vi "Moving Average.vi"(10 "Value":bool, 11 "Time Target (s)":dbl=0.25) -> (3 "Moving Boolean Average":bool)   [LabVIEW 2014]
uses:
  <vilib>/Analysis/baseanly.llb/Mean (DBL).vi
  <vilib>/Analysis/NI_AALBase.lvlib
panel:
  out "Elapsed Time (s)":dbl=0.3622617721557617
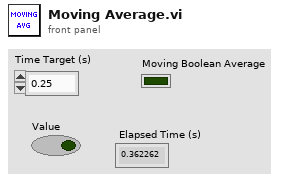
[diagram p1: front panel]
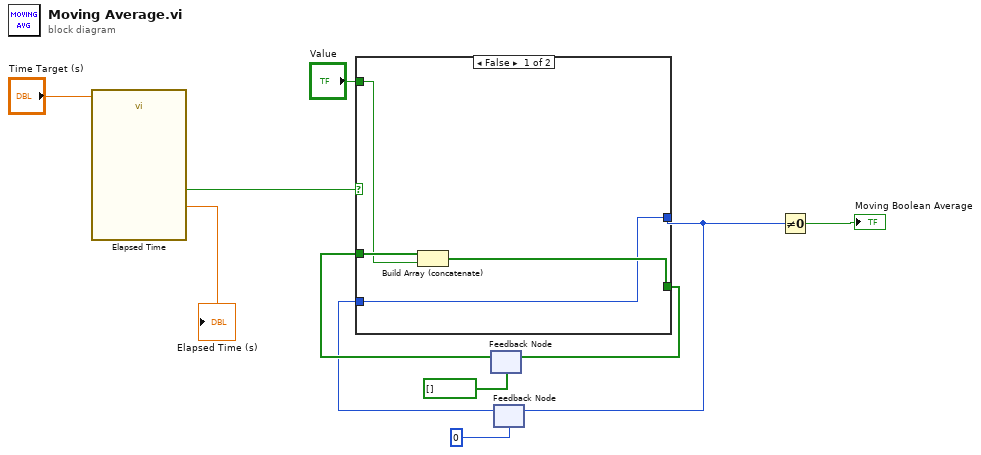
[diagram p0: block diagram]
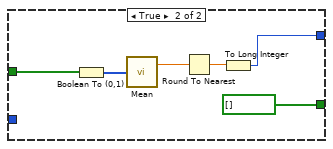
[diagram p2: hidden frame]
diagram:
  n1 = call "Elapsed Time"("Time Target (s)"="Time Target (s)") -> ("Elapsed Time (s)"=→"Elapsed Time (s)":dbl, "Time has Elapsed"=w10:bool)  [unwired: 11 in, 6 out]
  n2 = feedback #1(bool[] []) -> (w8:bool[])
  n3 = feedback #2(0) -> (w3:i32)
  n4 = case shown="False" w10 {
    tunnel: w8 -> [w14 w17]
    tunnel: "Value" -> [w13 _]
    tunnel: [w15 bool[] []] -> w9
    tunnel: [w12 w18] -> w2
    tunnel: w3 -> [w12 _]
    frame False {
      n5 = Build Array (concatenate)(w14, w13) -> (w15:bool[])
    }
    frame True {
      n6 = Boolean To (0,1)(Boolean=w17) -> (0, 1=w21:i16[])
      n7 = call-poly <vilib>:"Mean.vi"("X"=w21) -> ("mean"=w20:dbl)  [unwired: 1 out]
      n8 = Round To Nearest(number=w20) -> (nearest integer value=w19:dbl)
      n9 = To Long Integer(number=w19) -> (32bit integer=w18:i32)
    }
  }
  n10 = feedback-in #1(w9) -> ()
  n11 = feedback-in #2(w2) -> ()
  n12 = Not Equal To 0?(x=w2) -> (x != 0?=→"Moving Boolean Average":bool)
